vi "MapNumbers.vi"(0 "Input Variable":dbl, 5 "Input Minimum":dbl, 7 "Input Maximum":dbl, 9 "Output Minimum":dbl, 11 "Output Maximum":dbl) -> (4 "Output Variable":dbl)   [LabVIEW 2014]
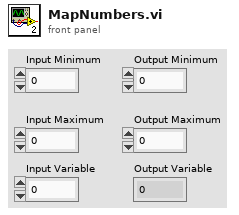
[diagram p1: front panel]
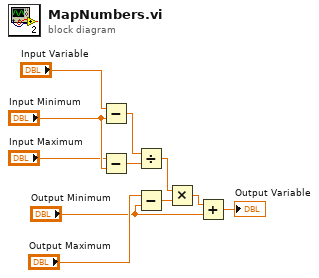
[diagram p0: block diagram]
diagram:
  n1 = Subtract(x="Input Variable", y="Input Minimum") -> (x-y=w8:dbl)
  n2 = Subtract(x="Input Maximum", y="Input Minimum") -> (x-y=w7:dbl)
  n3 = Divide(x=w8, y=w7) -> (x/y=w6:dbl)
  n4 = Subtract(x="Output Maximum", y="Output Minimum") -> (x-y=w5:dbl)
  n5 = Multiply(x=w6, y=w5) -> (x*y=w4:dbl)
  n6 = Add(x=w4, y="Output Minimum") -> (x+y=→"Output Variable":dbl)
